vi "Parse ERD Read Results (Rev 2 API).vi"(0 "Verify ERD Response?":bool=TRUE, 1 "Request ID":string, 2 "ERD Read Data In":T2 {"ERD Number" format="%.0x"}, 5 "Raw Message":string, 7 "Converted Data":T3 {"CRC" format="%04x"; "Length" format="%02x"; "Command" format="%02x"; "Destination" format="%02x"; "Source" format="%02x"}, 11 "Error In":errorcluster) -> (4 "Pass/Fail?":bool, 8 "ERD Read Data Out":T1 {"ERD Number" format="%.0x"}, 15 "Error Out":errorcluster)   [LabVIEW 2023, in "GEA2_Toolkit.lvlib"]
doc: "This VI takes the converted return data from the GEA2 Send and Receive and formats the Data based on the selections made in the Read ERD list. In addition, it also verifies the ERDs requested were returned."
uses:
  library/GEA2_Toolkit.lvlib
  type defs/Data Out.ctl
  type defs/ERD Read Data In.ctl
  type defs/ERD Read Data Out.ctl
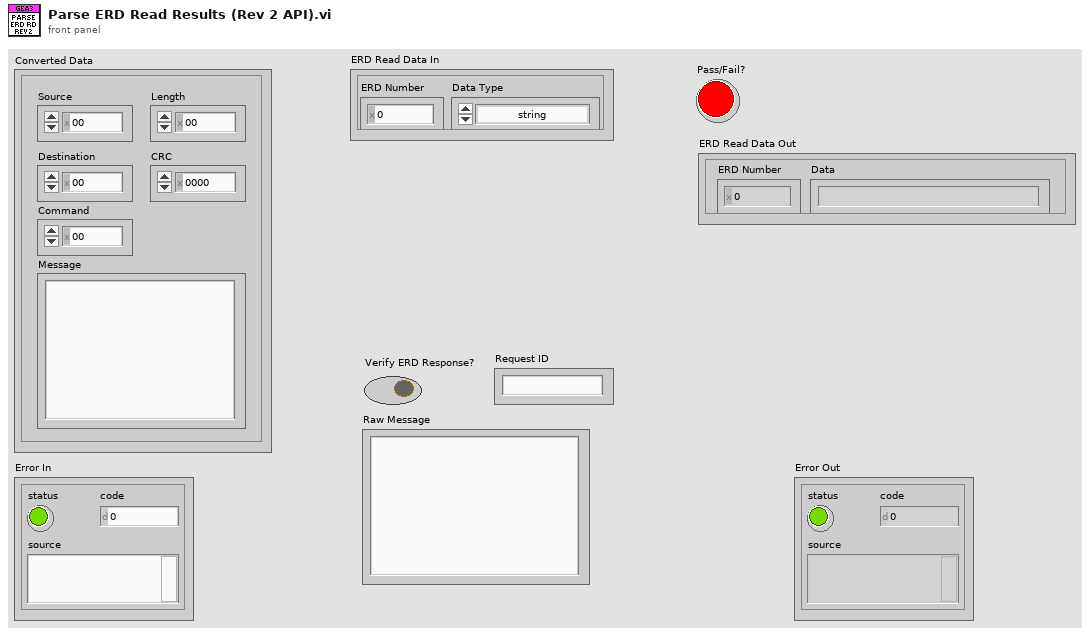
[diagram p1: front panel]
types:
  T1 = typedef "ERD Read Data Out.ctl" = cluster{"ERD Number":u16, "Data":string}
  T2 = typedef "ERD Read Data In.ctl" = cluster{"ERD Number":u16, "Data Type":enum16{"string", "boolean", "uint8_t", "uint16_t", "uint32_t", "uint64_t", "int8_t", "int16_t", "int32_t", "int64_t"}}
  T3 = typedef "GEA2_Toolkit.lvlib/Data Out.ctl" = cluster{"Source":u8, "Destination":u8, "Command":u8, "Length":u8, "CRC":u16, "Message":string}
  T4 = enum16{"string", "boolean", "uint8_t", "uint16_t", "uint32_t", "uint64_t", "int8_t", "int16_t", "int32_t", "int64_t"}
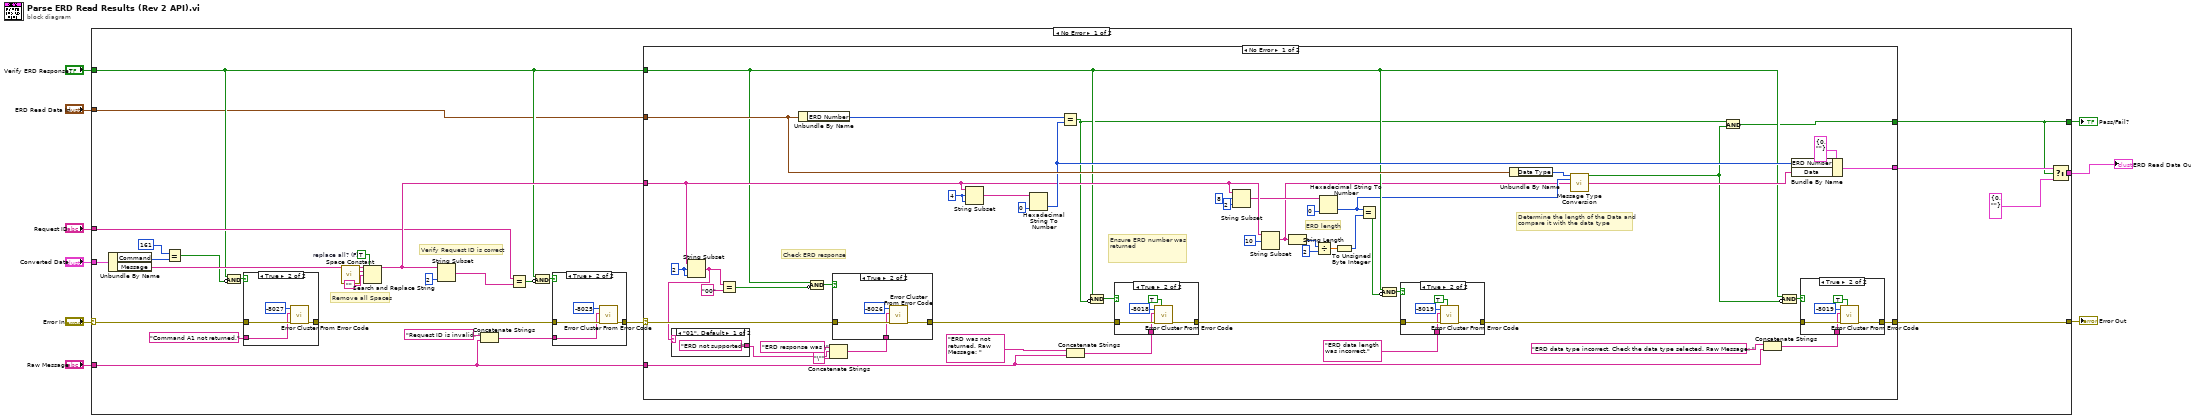
[diagram p0: block diagram]
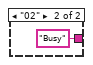
[diagram p5: hidden frame]
diagram:
  n1 = case shown="No Error" "Error In" {
    selector: "Error In" -> [w15 w125]
    tunnel: "Converted Data" -> [w38 _]
    tunnel: "ERD Read Data In" -> [w11 _]
    tunnel: [w20 _] -> w8
    tunnel: [w35 _] -> w1
    tunnel: [w29 w125] -> w6
    tunnel: "Raw Message" -> [w25 _]
    tunnel: "Verify ERD Response?" -> [w13 _]
    tunnel: "Request ID" -> [w22 _]
    frame No Error {
      w30 = TRUE  # replace all? (F)
      # "Remove all Spaces"
      # "Verify Request ID is correct"
      n2 = Unbundle By Name(w38) -> ("Command"=w19:u8, "Message"=w32:string)
      n3 = Equal?(x=u8 161, y=w19) -> (x = y?=w14:bool)
      n4 = Compound Arithmetic op=AND(w13, invert w14) -> (w17:bool)
      n5 = case shown="True" w17 {
        tunnel: [w39 w43] -> w16
        tunnel: w15 -> [w39 w41]
        tunnel: "Command A1 not returned." -> [_ w40]
        frame False {
        }
        frame True {
          n6 = call <vilib>:"Error Cluster From Error Code.vi"("error in (no error)"=w41, "error message (\"\")"=w40, "error code (0)"=-8027) -> ("error out"=w43:errorcluster)  [unwired: 6 in]
        }
      }
      n7 = call <vilib>:"Space Constant.vi"() -> ("String"=w34:string)
      n8 = Search and Replace String(replace all?=w30, input string=w32, search string=w34, replace string="") -> (result string=w31:string)  [unwired: 4 in, 3 out]
      n9 = String Subset(string=w31, length (rest)=2 ("length (rest)")) -> (substring=w21:string)  [unwired: 1 in]
      n10 = Concatenate Strings("Request ID is invalid. " ("string"), w25) -> (w27:string)
      n11 = Equal?(x=w22, y=w21) -> (x = y?=w24:bool)
      n12 = Compound Arithmetic op=AND(w13, invert w24) -> (w23:bool)
      n13 = case shown="True" w23 {
        tunnel: [w44 w48] -> w26
        tunnel: w16 -> [w44 w46]
        tunnel: w27 -> [_ w45]
        frame False {
        }
        frame True {
          n14 = call <vilib>:"Error Cluster From Error Code.vi"("error in (no error)"=w46, "error message (\"\")"=w45, "error code (0)"=-8025) -> ("error out"=w48:errorcluster)  [unwired: 6 in]
        }
      }
      n15 = case shown="No Error" w26 {
        selector: w26 -> [w79 w124]
        tunnel: [w50 _] -> w20
        tunnel: w31 -> [w67 _]
        tunnel: w11 -> [w98 _]
        tunnel: [w49 _] -> w36
        tunnel: [w97 w124] -> w29
        tunnel: w25 -> [w96 _]
        tunnel: w13 -> [w57 _]
        frame No Error {
          w82 = 2 ("offset (0)")
          w71 = u32 4
          # "ERD length"
          # "Check ERD response"
          # "Ensure ERD number was\nreturned"
          # "Determine the length of the Data and\ncompare it with the data type"
          n16 = String Subset(string=w67, offset (0)=w82, length (rest)=w82) -> (substring=w76:string)
          n17 = case shown="\"01\", Default" w76 {
            tunnel: ["ERD not supported" ("string") "Busy" ("string")] -> w74
            frame "01", Default {
            }
            frame "02" {
            }
          }
          n18 = Equal?(x=w76, y="00") -> (x = y?=w78:bool)
          n19 = Unbundle By Name(w98) -> ("ERD Number"=w93:u16)
          n20 = Compound Arithmetic op=AND(w57, invert w78) -> (w77:bool)
          n21 = Concatenate Strings("ERD response was \"" ("string"), w74, "\"" ("string")) -> (w73:string)
          n22 = case shown="True" w77 {
            tunnel: [w107 w109] -> w80
            tunnel: w79 -> [w107 w110]
            tunnel: w73 -> [_ w108]
            frame False {
            }
            frame True {
              n23 = call <vilib>:"Error Cluster From Error Code.vi"("error in (no error)"=w110, "error message (\"\")"=w108, "error code (0)"=-8026) -> ("error out"=w109:errorcluster)  [unwired: 6 in]
            }
          }
          n24 = String Subset(string=w67, offset (0)=w71, length (rest)=w71) -> (substring=w89:string)
          n25 = Hexadecimal String To Number(string=w89, default (0uL)=u16 0) -> (number=w92:u16)  [unwired: 1 in, 1 out]
          n26 = Equal?(x=w93, y=w92) -> (x = y?=w52:bool)
          n27 = Concatenate Strings("ERD was not returned. Raw Message: " ("string"), w96) -> (w86:string)
          n28 = Compound Arithmetic op=AND(w57, invert w52) -> (w84:bool)
          n29 = case shown="True" w84 {
            tunnel: [w112 w117] -> w60
            tunnel: w80 -> [w112 w116]
            tunnel: w86 -> [_ w113]
            frame False {
            }
            frame True {
              n30 = call <vilib>:"Error Cluster From Error Code.vi"("show call chain? (False)"=TRUE, "error in (no error)"=w116, "error message (\"\")"=w113, "error code (0)"=-8018) -> ("error out"=w117:errorcluster)  [unwired: 5 in]
            }
          }
          n31 = String Subset(string=w67, offset (0)=u32 8, length (rest)=2 ("length (rest)")) -> (substring=w66:string)
          n32 = String Subset(string=w67, offset (0)=u32 10) -> (substring=w53:string)  [unwired: 1 in]
          n33 = String Length(string=w53) -> (length=w64:i32)
          n34 = Divide(x=w64, y=2) -> (x/y=w62:dbl)
          n35 = Hexadecimal String To Number(string=w66, default (0uL)=u8 0 ("default (0 U32)")) -> (number=w54:u8)  [unwired: 1 in, 1 out]
          n36 = To Unsigned Byte Integer(number=w62) -> (unsigned 8bit integer=w61:u8)
          n37 = Equal?(x=w54, y=w61) -> (x = y?=w56:bool)
          n38 = Compound Arithmetic op=AND(w57, invert w56) -> (w58:bool)
          n39 = case shown="True" w58 {
            tunnel: [w99 w104] -> w59
            tunnel: w60 -> [w99 w103]
            tunnel: "ERD data length was incorrect." ("string") -> [_ w100]
            frame False {
            }
            frame True {
              n40 = call <vilib>:"Error Cluster From Error Code.vi"("show call chain? (False)"=TRUE, "error in (no error)"=w103, "error message (\"\")"=w100, "error code (0)"=-8019) -> ("error out"=w104:errorcluster)  [unwired: 5 in]
            }
          }
          n41 = Unbundle By Name(w98) -> ("Data Type"=w90:T4)
          n42 = call "Message Type Conversion.vi"("Data Type"=w90, "Data Length"=w54, "Message In"=w53) -> ("Pass/Fail?"=w51:bool, "Message Out"=w91:string)  [unwired: 11 in]
          n43 = Compound Arithmetic op=AND(w52, w51) -> (w50:bool)
          n44 = Concatenate Strings("ERD data type incorrect. Check the data type selected. Raw Message: " ("string"), w96) -> (w85:string)
          n45 = Compound Arithmetic op=AND(w57, invert w51) -> (w83:bool)
          n46 = Bundle By Name(cluster=T1 {"ERD Number"=0, "Data"=""} ("ERD Output"), "ERD Number"=w92, "Data"=w91) -> (w49:T1)
          n47 = case shown="True" w83 {
            tunnel: [w118 w123] -> w97
            tunnel: w59 -> [w118 w122]
            tunnel: w85 -> [_ w119]
            frame False {
            }
            frame True {
              n48 = call <vilib>:"Error Cluster From Error Code.vi"("show call chain? (False)"=TRUE, "error in (no error)"=w122, "error message (\"\")"=w119, "error code (0)"=-8019) -> ("error out"=w123:errorcluster)  [unwired: 5 in]
            }
          }
        }
        frame Error {
        }
      }
      n49 = Select(t=w36, s=w20, f=T1 {"ERD Number"=0, "Data"=""} ("ERD Output")) -> (s? t:f=w35:T1)
    }
    frame Error {
    }
  }
  "Pass/Fail?" <- w8
  "Error Out" <- w6
  "ERD Read Data Out" <- w1
